vi "VI5.vi"() -> ()   [LabVIEW 2010]
panel:
  in  "Porta_aux_torno 2":bool
  in  "Porta_aux_torno 1":bool
  in  "AS_RS Ativado":bool
  in  "Elevar Z":bool
  in  "ARMAZEM_PEGAR":bool
  in  "ESTEIRA_PEGAR":bool
  out "YD3":dbl
  out "YD2":dbl
  out "YD1":dbl
  out "YD0":dbl
  in  "Coordenada_Y":dbl min=0.0 max=2.0
  out "Z_Pos_Ok":bool
  out "Y_Pos_Ok":bool
  out "X_Pos_Ok":bool
  out "Z_Home_Ok":bool
  out "Y_Home_Ok":bool
  out "X_Home_Ok":bool
  in  "Z_CTRG":bool
  in  "Y_CTRG":bool
  in  "X_CTRG":bool
  in  "Z_HOME":bool
  in  "Y_HOME":bool
  in  "X_HOME":bool
  in  "Start":bool
  in  "Confirmação da posição":bool
  out "ZD3":dbl
  out "ZD2":dbl
  out "ZD1":dbl
  out "ZD0":dbl
  out "XD3":dbl
  out "XD2":dbl
  out "XD1":dbl
  out "XD0":dbl
  in  "Coordenada_Z":dbl min=0.0 max=12.0
  in  "Coordenada_X":dbl min=0.0 max=6.0
  out "Esteira 4":bool
  out "Esteira 3":bool
  out "Esteira 2":bool
  out "Esteira 1":bool
  in  "Eletroválvula 4":bool
  in  "Eletroválvula 3":bool
  in  "Eletroválvula 2":bool
  in  "Eletroválvula 1":bool
  out "Sensor 4":bool
  out "Sensor 3":bool
  out "Sensor 2":bool
  out "Sensor 1":bool
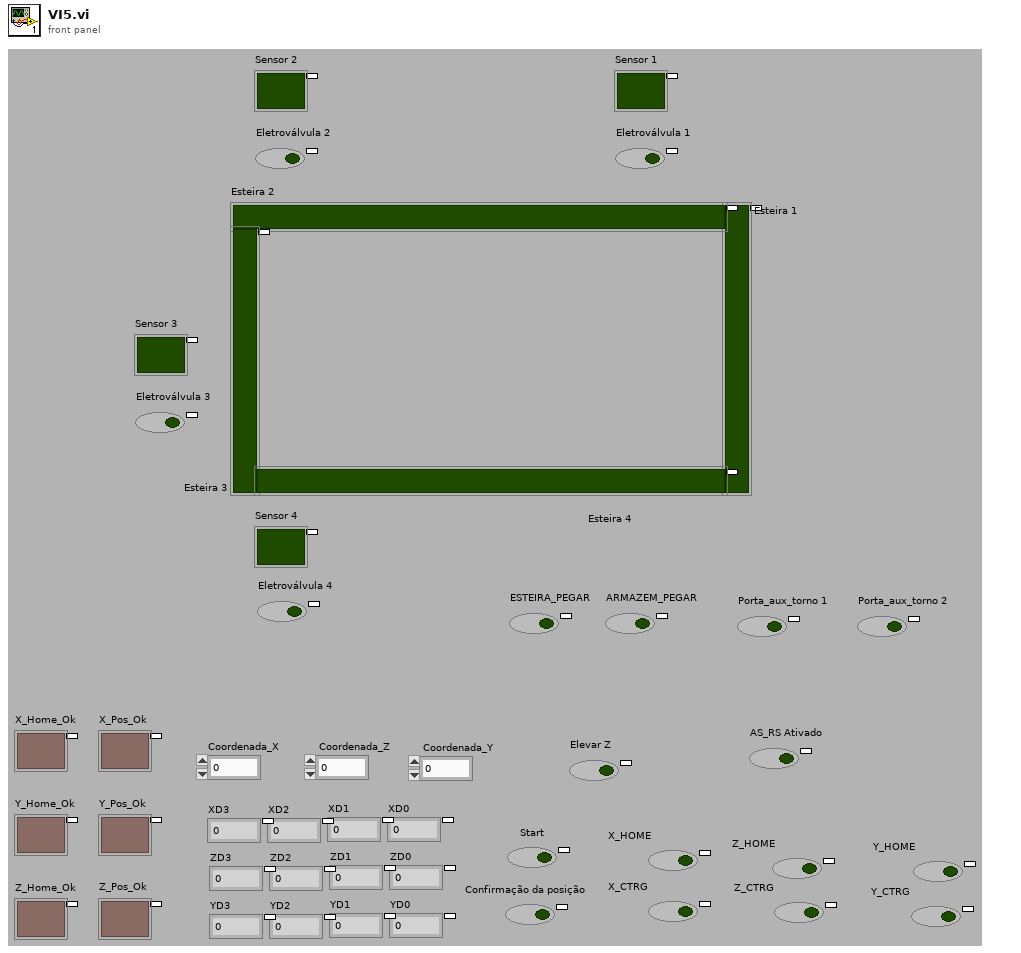
[diagram p1: front panel]
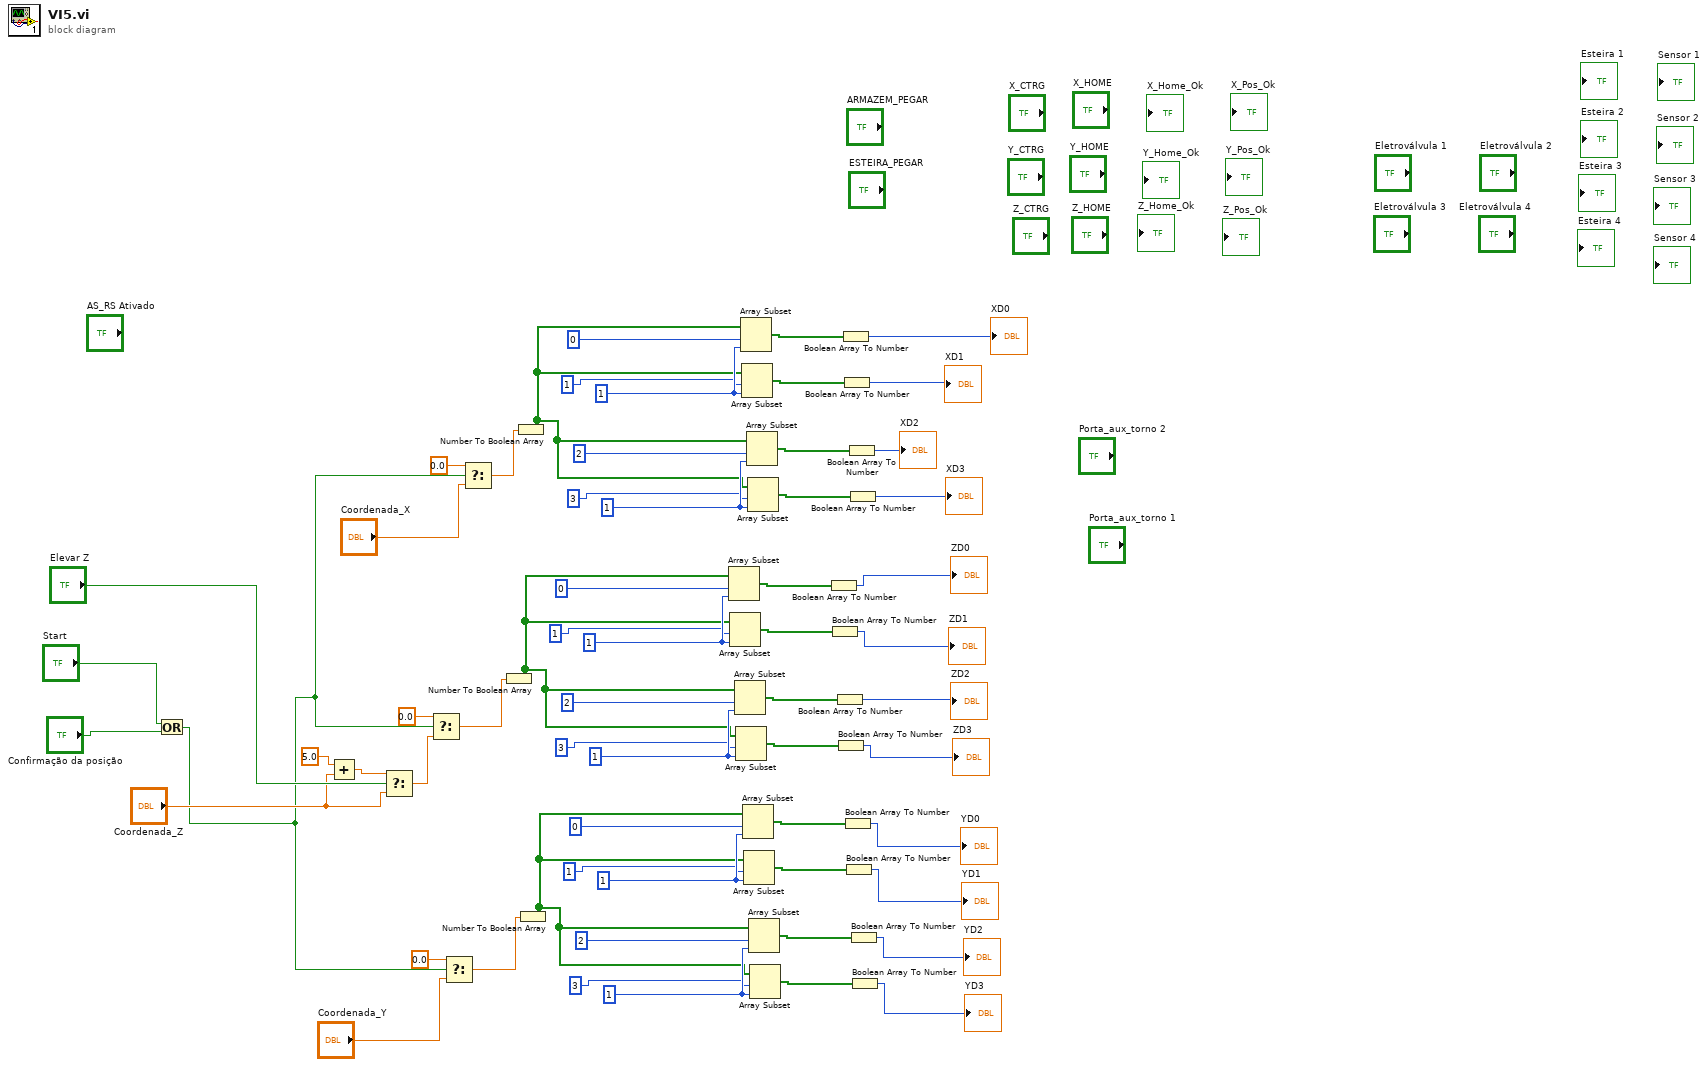
[diagram p0: block diagram]
diagram:
  w23 = 1 ("index")
  w28 = 1 ("index")
  w38 = 1 ("index")
  w43 = 1 ("index")
  w53 = 1 ("index")
  w58 = 1 ("index")
  n1 = Or(x="Start", y="Confirmação da posição") -> (x .or. y?=w1:bool)
  n2 = Add(x=5.0, y="Coordenada_Z") -> (x+y=w5:dbl)
  n3 = Select(t=w5, s="Elevar Z", f="Coordenada_Z") -> (s? t:f=w4:dbl)
  n4 = Select(t=0.0, s=w1, f=w4) -> (s? t:f=w11:dbl)
  n5 = Select(t=0.0, s=w1, f="Coordenada_Y") -> (s? t:f=w9:dbl)
  n6 = Select(t=0.0, s=w1, f="Coordenada_X") -> (s? t:f=w13:dbl)
  n7 = Number To Boolean Array(number=w11) -> (Boolean array=w36:bool[])
  n8 = Number To Boolean Array(number=w13) -> (Boolean array=w51:bool[])
  n9 = Number To Boolean Array(number=w9) -> (Boolean array=w21:bool[])
  n10 = Array Subset(array=w36, index=0, length=w43) -> (w46:bool[])
  n11 = Array Subset(array=w36, index=1, length=w43) -> (w44:bool[])
  n12 = Array Subset(array=w36, index=2, length=w38) -> (w41:bool[])
  n13 = Array Subset(array=w36, index=3, length=w38) -> (w39:bool[])
  n14 = Array Subset(array=w51, index=0, length=w58) -> (w61:bool[])
  n15 = Array Subset(array=w51, index=1, length=w58) -> (w59:bool[])
  n16 = Array Subset(array=w21, index=0, length=w28) -> (w31:bool[])
  n17 = Array Subset(array=w21, index=1, length=w28) -> (w29:bool[])
  n18 = Array Subset(array=w51, index=2, length=w53) -> (w56:bool[])
  n19 = Array Subset(array=w51, index=3, length=w53) -> (w54:bool[])
  n20 = Array Subset(array=w21, index=2, length=w23) -> (w26:bool[])
  n21 = Array Subset(array=w21, index=3, length=w23) -> (w24:bool[])
  n22 = Boolean Array To Number(Boolean array=w46) -> (number=→"ZD0":u32)
  n23 = Boolean Array To Number(Boolean array=w44) -> (number=→"ZD1":u32)
  n24 = Boolean Array To Number(Boolean array=w41) -> (number=→"ZD2":u32)
  n25 = Boolean Array To Number(Boolean array=w39) -> (number=→"ZD3":u32)
  n26 = Boolean Array To Number(Boolean array=w61) -> (number=→"XD0":u32)
  n27 = Boolean Array To Number(Boolean array=w59) -> (number=→"XD1":u32)
  n28 = Boolean Array To Number(Boolean array=w31) -> (number=→"YD0":u32)
  n29 = Boolean Array To Number(Boolean array=w29) -> (number=→"YD1":u32)
  n30 = Boolean Array To Number(Boolean array=w56) -> (number=→"XD2":u32)
  n31 = Boolean Array To Number(Boolean array=w54) -> (number=→"XD3":u32)
  n32 = Boolean Array To Number(Boolean array=w26) -> (number=→"YD2":u32)
  n33 = Boolean Array To Number(Boolean array=w24) -> (number=→"YD3":u32)
